vi "Move.vi"(8 "error in (no error)":errorcluster, 10 "Move Data":cluster{"Direction":T1, "Step (px)":u16}, 11 "Geometric Figure in":refnum<class "Ghosts.lvclass">) -> (0 "error out":errorcluster, 3 "Geometric Figure out":refnum<class "Ghosts.lvclass">)   [LabVIEW 2016, in "PacManClasses.lvlib" / "Ghosts.lvclass"]
uses:
  Ghosts.lvclass
  Generic Controls/Direction.ctl
  Geometric Figure/UI Object.lvclass
  PacManClasses.lvlib
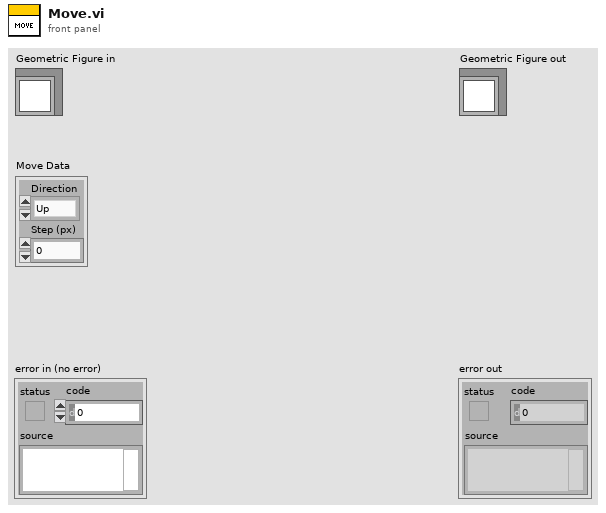
[diagram p1: front panel]
types:
  T1 = typedef "PacManClasses.lvlib/Direction.ctl" = enum16{"Up", "Down", "Left", "Right"}
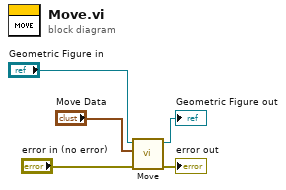
[diagram p0: block diagram]
diagram:
  n1 = call-parent "Move.vi"("error in (no error)"="error in (no error)", "Move Data"="Move Data", "Geometric Figure in"="Geometric Figure in") -> ("error out"=→"error out":errorcluster, "Geometric Figure out"=→"Geometric Figure out":refnum<class "Ghosts.lvclass">)  [unwired: 7 in]
